vi "practica2.vi"() -> ()   [LabVIEW 2016]
uses:
  <vilib>/DAQmx/read.llb/DAQmx Read (Analog 1D DBL NChan 1Samp).vi
  <vilib>/DAQmx/create/channels.llb/DAQmx Create Channel (AI-Voltage-Basic).vi
  <vilib>/DAQmx/configure/timing.llb/DAQmx Timing (Sample Clock).vi
  <vilib>/DAQmx/miscellaneous.llb/DAQmx Fill In Error Info.vi
panel:
  in  "Stop Button":bool
  out "XY Graph":cluster{dbl[], dbl[]}(graph)
  in  "L 3":dbl(slide) scale=0.0..3.0
  in  "L 2":dbl(slide) scale=0.0..3.0
  in  "L 1":dbl(slide) scale=0.0..3.0
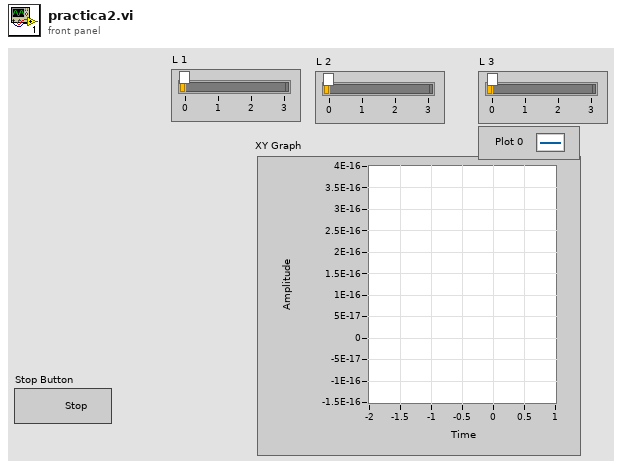
[diagram p1: front panel]
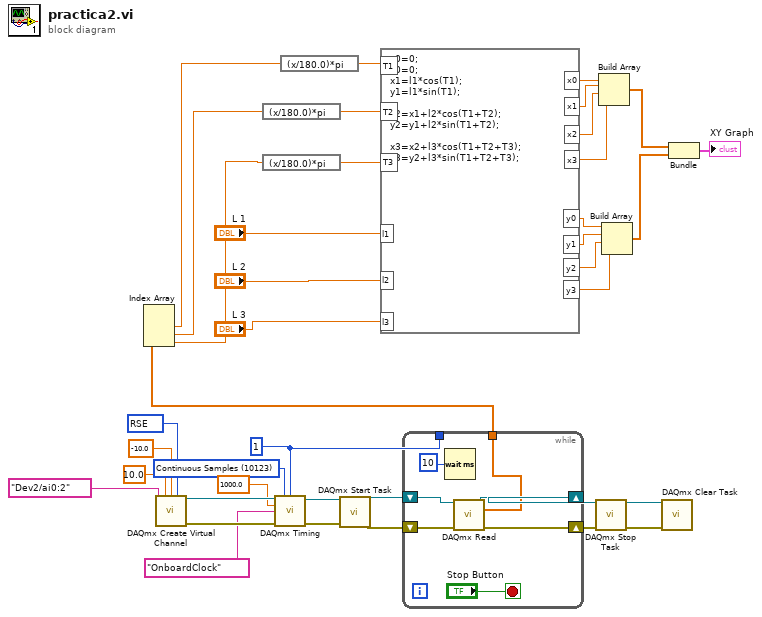
[diagram p0: block diagram]
diagram:
  w11 = 1 ("samples per channel")
  w18 = 10123 items=["Finite Samples"=10178, "Continuous Samples"=10123, "Hardware Timed Single Point"=12522] ("sample mode")
  w21 = 10083 items=["Default"=-1, "RSE"=10083, "NRSE"=10078, "Differential"=10106, "Pseudodifferential"=12529] ("input terminal configuration")
  n1 = call-poly <vilib>:"DAQmx Create Virtual Channel.vi"("maximum value"=10.0, "minimum value"=-10.0, "input terminal configuration"=w21, "physical channels"=tag "Dev2/ai0:2") -> ("task out"=w20:refnum<k21>, "error out"=w19:errorcluster)  [unwired: 10 in]
  n2 = call-poly <vilib>:"DAQmx Timing.vi"("task/channels in"=w20, "sample mode"=w18, "samples per channel"=w11, "rate"=1000.0, "source"=tag "OnboardClock", "error in"=w19) -> ("task out"=w15:refnum<k21>, "error out"=w14:errorcluster)  [unwired: 8 in]
  n3 = call <vilib>:"DAQmx Start Task.vi"("task/channels in"=w15, "error in"=w14) -> ("task out"=w13:refnum<k21>, "error out"=w12:errorcluster)  [unwired: 12 in]
  n4 = while {
    tunnel: w11 -> [_]
    shift-right: [w44] -> w10
    shift-left: w13 -> [w46]
    shift-right: [w43] -> w9
    shift-left: w12 -> [w45]
    tunnel: [w40] -> w6
    stop <- "Stop Button" stop-if-true
    n5 = Wait (ms)(milliseconds to wait=u32 10) -> ()  [unwired: 1 out]
    n6 = call-poly <vilib>:"DAQmx Read.vi"("task/channels in"=w46, "error in"=w45) -> ("task out"=w44:refnum<k21>, "data"=w40:dbl[], "error out"=w43:errorcluster)  [unwired: 11 in]
  }
  n7 = Index Array(array=w6) -> (element #1=w3:dbl, element #2=w2:dbl, element #3=w1:dbl)  [unwired: 3 in]
  n8 = expression code="(x/180.0)*pi" ("degrees to radians")(w2) -> (w38:dbl)
  n9 = expression code="(x/180.0)*pi" ("degrees to radians")(w1) -> (w31:dbl)
  n10 = expression code="(x/180.0)*pi" ("degrees to radians")(w3) -> (w4:dbl)
  n11 = formula code="x0=0;\ny0=0;\nx1=l1*cos(T1);\ny1=l1*sin(T1);\n\nx2=x1+l2*cos(T1+T2);\ny2=y1+l2*sin(T1+T2);\n\nx3=x2+l3*cos(T1+T2+T3);\ny3=y2+l3*sin(T1+T2+T3);"("T1"=w4, "l1"="L 1", "T2"=w38, "T3"=w31, "l2"="L 2", "l3"="L 3") -> ("x0"=w37:dbl, "x1"=w36:dbl, "y0"=w35:dbl, "y1"=w34:dbl, "x2"=w30:dbl, "y2"=w29:dbl, "y3"=w26:dbl, "x3"=w25:dbl)
  n12 = call <vilib>:"DAQmx Stop Task.vi"("task/channels in"=w10, "error in"=w9) -> ("task out"=w8:refnum<k21>, "error out"=w7:errorcluster)  [unwired: 12 in]
  n13 = Build Array(w37, w36, w30, w25) -> (w33:dbl[])
  n14 = Build Array(w35, w34, w29, w26) -> (w32:dbl[])
  n15 = call <vilib>:"DAQmx Clear Task.vi"("task in"=w8, "error in"=w7) -> ()  [unwired: 13 in, 1 out]
  n16 = Bundle(w33, w32) -> (→"XY Graph":cluster{dbl[], dbl[]})  [unwired: 1 in]
